vi "Write Data(IL).vi"(8 "error in (no error)":errorcluster, 9 "NAD":u8, 10 "Tx Msg":u8[][](array[numeric]), 11 "LIN Device in":T1={"Master Frame(3C)"="MasterReq\nSPA3414_ConfigurationsCMAGeely_CEMCALYPSOSDB34XX0Cfg_LIN3_190709_", "Slave Frame(3D)"="SlaveResp\nSPA3414_ConfigurationsCMAGeely_CEMCALYPSOSDB34XX0Cfg_LIN3_190709_", "Request Schedule"="CEMLIN3DiagRequestSchedule\nSPA3414_ConfigurationsCMAGeely_CEMCALYPSOSDB34XX0Cfg_LIN3_190709_", "Response Schedule"="CEMLIN3DiagResponseSchedule\nSPA3414_ConfigurationsCMAGeely_CEMCALYPSOSDB34XX0Cfg_LIN3_190709_", "Frame Write SCU"="", "Frame Read SCU"="", "LIN Name"=""}) -> (0 "error out":errorcluster, 2 "Array":u8[](array[numeric]), 3 "LIN Device out":T1={"Master Frame(3C)"="MasterReq\nSPA3414_ConfigurationsCMAGeely_CEMCALYPSOSDB34XX0Cfg_LIN3_190709_", "Slave Frame(3D)"="SlaveResp\nSPA3414_ConfigurationsCMAGeely_CEMCALYPSOSDB34XX0Cfg_LIN3_190709_", "Request Schedule"="CEMLIN3DiagRequestSchedule\nSPA3414_ConfigurationsCMAGeely_CEMCALYPSOSDB34XX0Cfg_LIN3_190709_", "Response Schedule"="CEMLIN3DiagResponseSchedule\nSPA3414_ConfigurationsCMAGeely_CEMCALYPSOSDB34XX0Cfg_LIN3_190709_", "Frame Write SCU"="", "Frame Read SCU"="", "LIN Name"=""})   [LabVIEW 2018]
uses:
  LIN Device.ctl
  <vilib>/xnet/xnet.llb/XNET Frame LIN.ctl
  <vilib>/xnet/xnet.llb/XNET Frame Type LIN.ctl
  <vilib>/xnet/xnet.llb/XNET Write (State LIN Schedule Change).vi
  <vilib>/xnet/xnet.llb/XNET Write (Frame LIN).vi
  <vilib>/xnet/xnet.llb/XNET Wait (Transmit Complete).vi
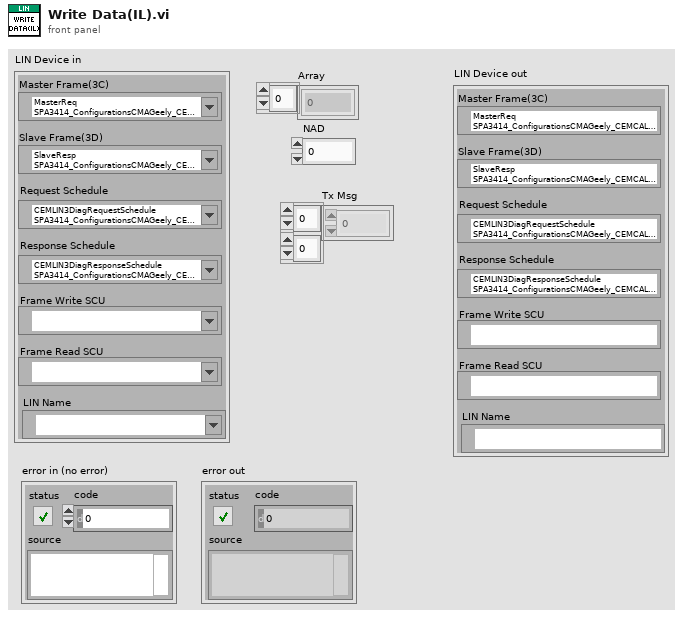
[diagram p1: front panel]
types:
  T1 = typedef "LIN Device.ctl" = cluster{"Master Frame(3C)":refnum<k21>, "Slave Frame(3D)":refnum<k21>, "Request Schedule":refnum<k21>, "Response Schedule":refnum<k21>, "Frame Write SCU":refnum<k21>, "Frame Read SCU":refnum<k21>, "LIN Name":refnum<k21>}
  T2 = typedef "XNET Frame LIN.ctl" = cluster{"timestamp":timestamp, "payload":u8[], "identifier":u32, "type":T3, "event ID":u8, "event slot?":bool, "echo?":bool}
  T3 = typedef "XNET Frame Type LIN.ctl" = u8
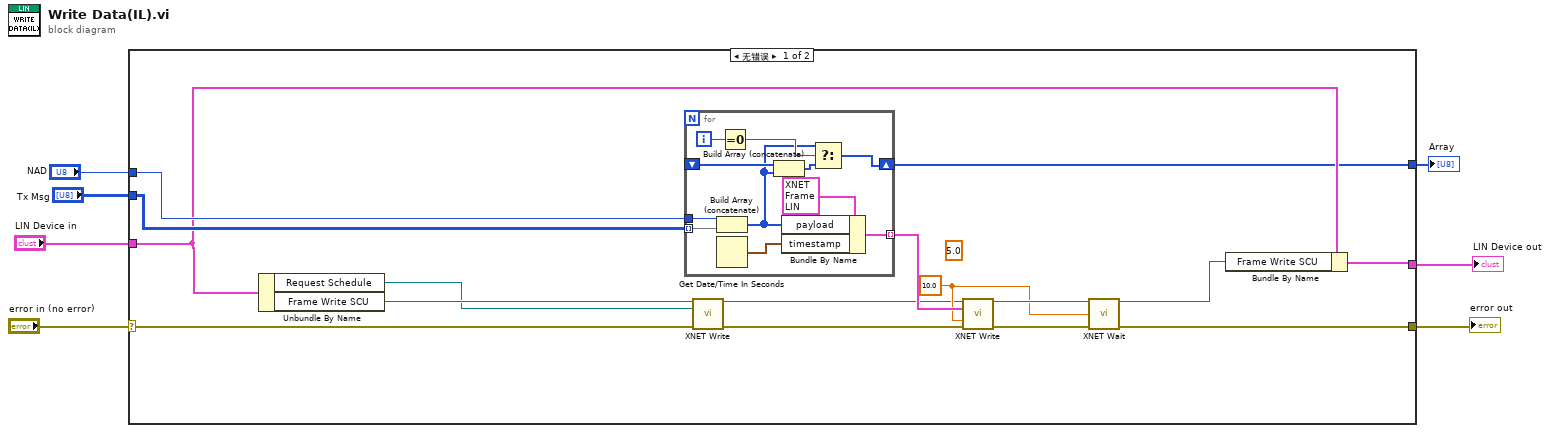
[diagram p0: block diagram]
diagram:
  n1 = case shown="无错误" "error in (no error)" {
    selector: "error in (no error)" -> [w10 w36]
    tunnel: "LIN Device in" -> [w17 w35]
    tunnel: "Tx Msg" -> [w23 _]
    tunnel: "NAD" -> [w22 _]
    tunnel: [w13 w36] -> w4
    tunnel: [w16 w35] -> w1
    tunnel: [w15 _] -> w3
    frame No Error {
      (unwired) 5.0 ("timeout (10)")
      w18 = 10.0 ("timeout (10)")
      n2 = Unbundle By Name(w17) -> ("Request Schedule"=w11:refnum<k21>, "Frame Write SCU"=w12:refnum<k21>)
      n3 = for {
        tunnel: w23 -> [w33] mode=indexing
        tunnel: w22 -> [w34]
        tunnel: [w28] -> w21 mode=indexing
        shift-right: [w27] -> w15
        shift-left: _ -> [w26]
        i -> [w30]
        n4 = Build Array (concatenate)(w34, w33) -> (w25:u8[])
        n5 = Get Date/Time In Seconds() -> (seconds since 1Jan1904=w31:timestamp)
        n6 = Equal To 0?(x=w30) -> (x = 0?=w29:bool)
        n7 = Build Array (concatenate)(w26, w25) -> (w24:u8[])
        n8 = Bundle By Name(cluster=T2 {"timestamp"=timestamp(0 s since 1904-01-01), "payload"=[], "identifier"=60, "type"=64, "event ID"=0, "event slot?"=FALSE, "echo?"=FALSE} ("LIN frame"), "payload"=w25, "timestamp"=w31) -> (w28:T2)
        n9 = Select(t=w25, s=w29, f=w24) -> (s? t:f=w27:u8[])
      }
      n10 = call-poly <vilib>:"XNET Write.vi"("session in"=w12, "data"=w11, "error in (no error)"=w10) -> ("session out"=w8:refnum<k21>, "error out"=w9:errorcluster)  [unwired: 11 in]
      n11 = call-poly <vilib>:"XNET Write.vi"("session in"=w8, "data"=w21, "timeout (10)"=w18, "error in (no error)"=w9) -> ("session out"=w19:refnum<k21>, "error out"=w20:errorcluster)  [unwired: 10 in]
      n12 = call-poly <vilib>:"XNET Wait.vi"("session in"=w19, "timeout (10)"=w18, "error in (no error)"=w20) -> ("session out"=w14:refnum<k21>, "error out"=w13:errorcluster)  [unwired: 11 in]
      n13 = Bundle By Name(cluster=w17, "Frame Write SCU"=w14) -> (w16:T1)
    }
    frame Error {
    }
  }
  "error out" <- w4
  "Array" <- w3
  "LIN Device out" <- w1
